vi "SelectOPCTags.HandleSymbolSelection.vi"(7 "This VI":refnum<vi>, 8 "error in":errorcluster, 10 "Tag":string, 11 "CtlRef":refnum<vi>) -> (0 "error out":errorcluster)   [LabVIEW 2015, in "OPC UA Client System Explorer.lvlib"]
uses:
  OPC UA Client System Explorer.lvlib
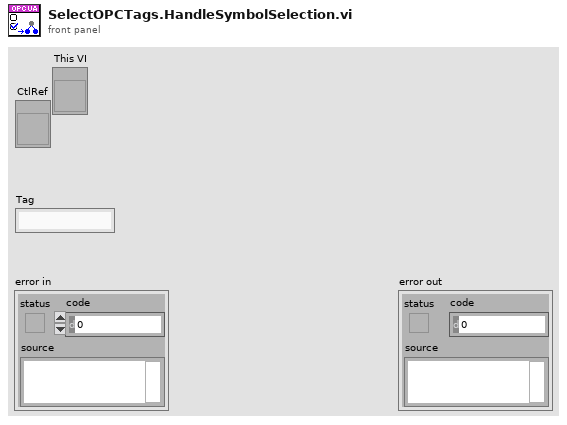
[diagram p1: front panel]
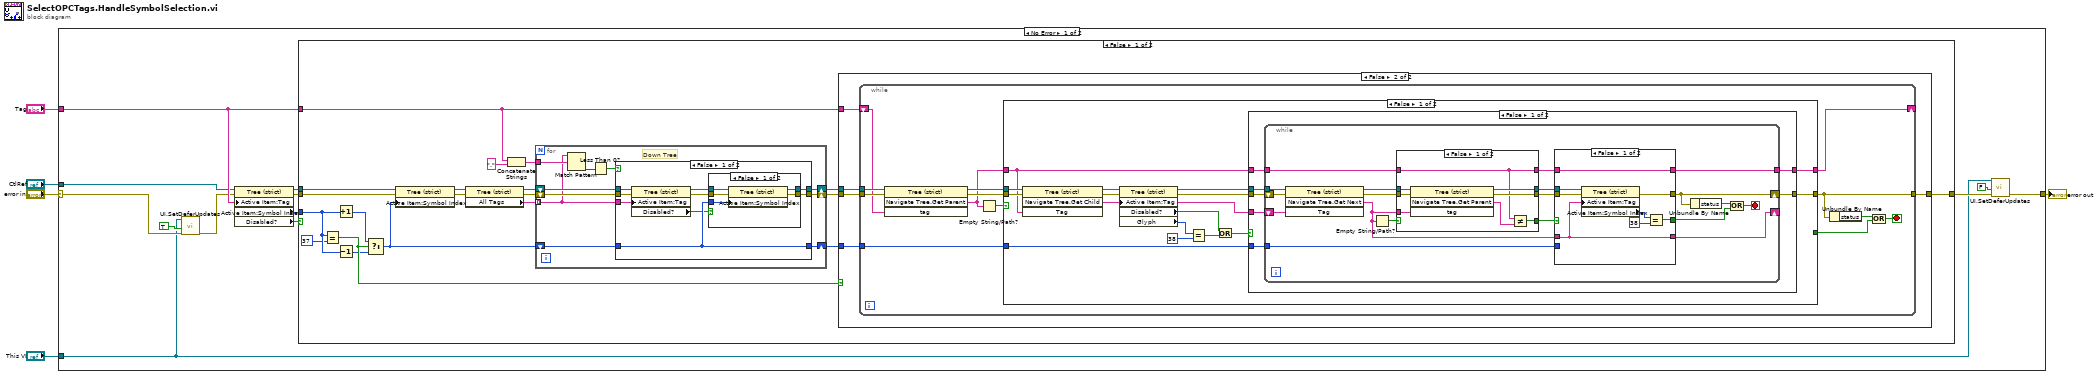
[diagram p0: block diagram]
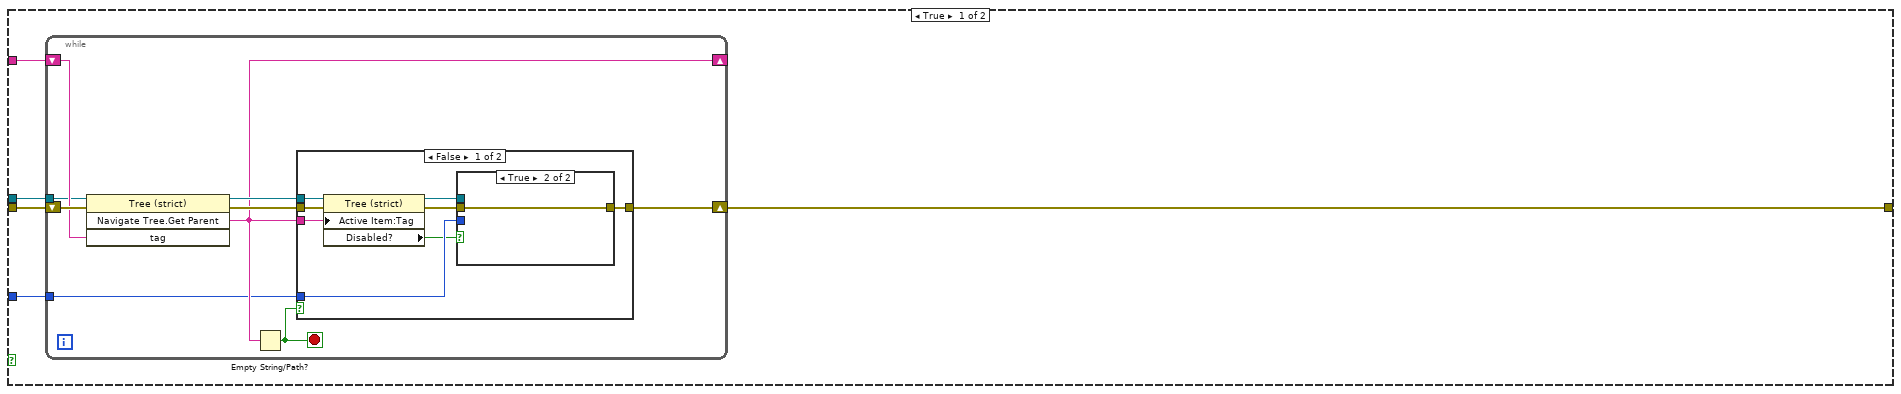
[diagram p2: hidden frame]
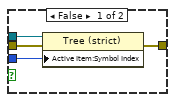
[diagram p3: hidden frame]
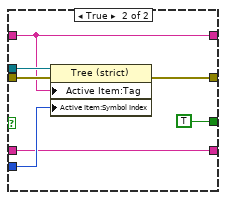
[diagram p6: hidden frame]
diagram:
  n1 = case shown="No Error" "error in" {
    selector: "error in" -> [w11 w189]
    tunnel: [w8 w189] -> w5
    tunnel: "Tag" -> [w18 _]
    tunnel: "CtlRef" -> [w17 _]
    tunnel: "This VI" -> [w6 _]
    frame No Error {
      n2 = call "UI.SetDeferUpdates.vi"("error in (no error)"=w11, "Defer Panel Updates"=TRUE, "This VI"=w6) -> ("error out"=w10:errorcluster)  [unwired: 8 in]
      n3 = property class="Tree (strict)"(reference=w17, error in=w10, "Active Item:Tag"=w18) -> (reference out=w15:refnum<vi>, error out=w16:errorcluster, "Active Item:Symbol Index"=w14:i32, "Disabled?"=w13:bool)
      n4 = case shown="False" w13 {
        tunnel: [w37 w188] -> w7
        tunnel: w18 -> [w35 _]
        tunnel: w16 -> [w24 w188]
        tunnel: w15 -> [w23 _]
        tunnel: w14 -> [w21 _]
        frame False {
          n5 = Equal?(x=w21, y=37 ("Active Item:Symbol Index")) -> (x = y?=w32:bool)
          n6 = Increment(x=w21) -> (x+1=w20:i32)
          n7 = Decrement(x=w21) -> (x-1=w22:i32)
          n8 = Select(t=w20, s=w32, f=w22) -> (s? t:f=w33:i32)
          n9 = property class="Tree (strict)"(reference=w23, error in=w24, "Active Item:Symbol Index"=w33) -> (reference out=w25:refnum<vi>, error out=w26:errorcluster)
          n10 = property class="Tree (strict)"(reference=w25, error in=w26) -> (reference out=w28:refnum<vi>, error out=w27:errorcluster, "All Tags"=w31:string[])
          n11 = Concatenate Strings(w35, "." ("string")) -> (w30:string)
          n12 = for {
            tunnel: w30 -> [w168]
            tunnel: w31 -> [w161] mode=indexing
            shift-right: [w164] -> w34
            shift-left: w27 -> [w163]
            shift-right: [w160] -> w36
            shift-left: w28 -> [w162]
            shift-right: [w159] -> w38
            shift-left: w33 -> [w165]
            # "Down Tree"
            n13 = Match Pattern(string=w161, regular expression=w168) -> (offset past match=w167:i32)  [unwired: 1 in, 3 out]
            n14 = Less Than 0?(x=w167) -> (x < 0?=w166:bool)
            n15 = case shown="False" w166 {
              tunnel: w163 -> [w176 w187]
              tunnel: w162 -> [w177 w186]
              tunnel: w161 -> [w175 _]
              tunnel: w165 -> [w170 w185]
              tunnel: [w171 w187] -> w164
              tunnel: [w172 w186] -> w160
              tunnel: [w170 w185] -> w159
              frame False {
                n16 = property class="Tree (strict)"(reference=w177, error in=w176, "Active Item:Tag"=w175) -> (reference out=w173:refnum<vi>, error out=w174:errorcluster, "Disabled?"=w169:bool)
                n17 = case shown="False" w169 {
                  tunnel: w174 -> [w182 w183]
                  tunnel: w173 -> [w181 w184]
                  tunnel: [w180 w184] -> w172
                  tunnel: [w179 w183] -> w171
                  tunnel: w170 -> [w178 _]
                  frame False {
                    n18 = property class="Tree (strict)"(reference=w181, error in=w182, "Active Item:Symbol Index"=w178) -> (reference out=w180:refnum<vi>, error out=w179:errorcluster)
                  }
                  frame True {
                  }
                }
              }
              frame True {
              }
            }
          }
          n19 = case shown="False" w32 {
            tunnel: w34 -> [w43 w70]
            tunnel: w35 -> [w42 w68]
            tunnel: w36 -> [w41 w69]
            tunnel: [w40 w71] -> w37
            tunnel: w38 -> [w39 w67]
            frame True {
              n20 = while {
                tunnel: w41 -> [w50]
                shift-right: [w45] -> w40
                shift-left: w43 -> [w52]
                shift-right: [w47] -> _
                shift-left: w42 -> [w51]
                tunnel: w39 -> [w46]
                stop <- w44 stop-if-true
                n21 = invoke on="Invoke Node" class="Tree (strict)" method="Navigate Tree.Get Parent"(reference=w50, error in=w52, "tag"=w51) -> (reference out=w49:refnum<vi>, error out=w48:errorcluster, "Navigate Tree:Get Parent"=w47:string)  [unwired: 1 in, 1 out]
                n22 = Empty String/Path?(string/path=w47) -> (empty?=w44:bool)
                n23 = case shown="False" w44 {
                  tunnel: w48 -> [w59 w66]
                  tunnel: w49 -> [w60 _]
                  tunnel: w47 -> [w58 _]
                  tunnel: w46 -> [w54 _]
                  tunnel: [w55 w66] -> w45
                  frame False {
                    n24 = property class="Tree (strict)"(reference=w60, error in=w59, "Active Item:Tag"=w58) -> (reference out=w56:refnum<vi>, error out=w57:errorcluster, "Disabled?"=w53:bool)
                    n25 = case shown="True" w53 {
                      tunnel: w57 -> [w64 w65]
                      tunnel: w56 -> [w63 _]
                      tunnel: [w62 w65] -> w55
                      tunnel: w54 -> [w61 _]
                      frame False {
                        n26 = property class="Tree (strict)"(reference=w63, error in=w64, "Active Item:Symbol Index"=w61) -> (error out=w62:errorcluster)  [unwired: 1 out]
                      }
                      frame True {
                      }
                    }
                  }
                  frame True {
                  }
                }
              }
            }
            frame False {
              n27 = while {
                tunnel: [w75] -> w71
                tunnel: w70 -> [w84]
                tunnel: w69 -> [w83]
                shift-right: [w78] -> _
                shift-left: w68 -> [w77]
                tunnel: w67 -> [w76]
                stop <- w73 stop-if-true
                n28 = invoke on="Invoke Node" class="Tree (strict)" method="Navigate Tree.Get Parent"(reference=w83, error in=w84, "tag"=w77) -> (reference out=w81:refnum<vi>, error out=w82:errorcluster, "Navigate Tree:Get Parent"=w80:string)  [unwired: 1 in, 1 out]
                n29 = Empty String/Path?(string/path=w80) -> (empty?=w79:bool)
                n30 = case shown="False" w79 {
                  selector: w79 -> [_ w156]
                  tunnel: w76 -> [w100 _]
                  tunnel: [w99 w158] -> w75
                  tunnel: w82 -> [w98 w158]
                  tunnel: w81 -> [w97 _]
                  tunnel: w80 -> [w92 w157]
                  tunnel: [w90 w157] -> w78
                  tunnel: [_ w156] -> w72
                  frame False {
                    n31 = invoke on="Invoke Node" class="Tree (strict)" method="Navigate Tree.Get Child"(reference=w97, error in=w98, "Tag"=w92) -> (reference out=w96:refnum<vi>, error out=w94:errorcluster, "Navigate Tree:Get Child"=w85:string)  [unwired: 1 in, 1 out]
                    n32 = property class="Tree (strict)"(reference=w96, error in=w94, "Active Item:Tag"=w85) -> (reference out=w95:refnum<vi>, error out=w93:errorcluster, "Disabled?"=w88:bool, "Glyph"=w89:i32)
                    n33 = Equal?(x=w89, y=38 ("Active Item:Symbol Index")) -> (x = y?=w87:bool)
                    n34 = Or(x=w88, y=w87) -> (x .or. y?=w86:bool)
                    n35 = case shown="False" w86 {
                      tunnel: w100 -> [w107 _]
                      tunnel: [w106 w155] -> w99
                      tunnel: w95 -> [w105 _]
                      tunnel: w93 -> [w104 w155]
                      tunnel: w85 -> [w103 _]
                      tunnel: w92 -> [w102 w154]
                      tunnel: [w101 w154] -> w90
                      frame False {
                        n36 = while {
                          tunnel: w107 -> [w126]
                          tunnel: w105 -> [w123]
                          shift-right: [w113] -> w106
                          shift-left: w104 -> [w125]
                          shift-right: [w108] -> _
                          shift-left: w103 -> [w124]
                          tunnel: w102 -> [w114]
                          tunnel: [w109] -> w101
                          stop <- w111 stop-if-true
                          n37 = invoke on="Invoke Node" class="Tree (strict)" method="Navigate Tree.Get Next"(reference=w123, error in=w125, "Tag"=w124) -> (reference out=w122:refnum<vi>, error out=w120:errorcluster, "Navigate Tree:Get Next Item"=w115:string)  [unwired: 1 in, 1 out]
                          n38 = Empty String/Path?(string/path=w115) -> (empty?=w117:bool)
                          n39 = case shown="False" w117 {
                            selector: w117 -> [_ w138]
                            tunnel: w122 -> [w134 w136]
                            tunnel: [w133 w136] -> w121
                            tunnel: w120 -> [w132 w137]
                            tunnel: [w131 w137] -> w119
                            tunnel: [w129 w138] -> w118
                            tunnel: w114 -> [w127 w135]
                            tunnel: w115 -> [w128 _]
                            tunnel: [w127 w135] -> w116
                            frame False {
                              n40 = invoke on="Invoke Node" class="Tree (strict)" method="Navigate Tree.Get Parent"(reference=w134, error in=w132, "tag"=w128) -> (reference out=w133:refnum<vi>, error out=w131:errorcluster, "Navigate Tree:Get Parent"=w130:string)  [unwired: 1 in, 1 out]
                              n41 = Not Equal?(x=w127, y=w130) -> (x != y?=w129:bool)
                            }
                            frame True {
                            }
                          }
                          n42 = case shown="False" w118 {
                            tunnel: w126 -> [_ w149]
                            tunnel: w119 -> [w146 w151]
                            tunnel: [w141 w152] -> w113
                            tunnel: w121 -> [w145 w150]
                            tunnel: w115 -> [w139 w147]
                            tunnel: [w142 TRUE] -> w110
                            tunnel: w116 -> [w140 w148]
                            tunnel: [w140 w148] -> w109
                            tunnel: [w139 w147] -> w108
                            frame False {
                              n43 = property class="Tree (strict)"(reference=w145, error in=w146, "Active Item:Tag"=w139) -> (error out=w141:errorcluster, "Active Item:Symbol Index"=w143:i32)  [unwired: 1 out]
                              n44 = Equal?(x=w143, y=38 ("Active Item:Symbol Index")) -> (x = y?=w142:bool)
                            }
                            frame True {
                              n45 = property class="Tree (strict)"(reference=w150, error in=w151, "Active Item:Tag"=w148, "Active Item:Symbol Index"=w149) -> (error out=w152:errorcluster)  [unwired: 1 out]
                            }
                          }
                          n46 = Unbundle By Name(w113) -> ("status"=w112:bool)
                          n47 = Compound Arithmetic op=OR(w112, w110) -> (w111:bool)
                        }
                      }
                      frame True {
                      }
                    }
                  }
                  frame True {
                  }
                }
                n48 = Unbundle By Name(w75) -> ("status"=w74:bool)
                n49 = Compound Arithmetic op=OR(w74, w72) -> (w73:bool)
              }
            }
          }
        }
        frame True {
        }
      }
      n50 = call "UI.SetDeferUpdates.vi"("error in (no error)"=w7, "Defer Panel Updates"=FALSE, "This VI"=w6) -> ("error out"=w8:errorcluster)  [unwired: 8 in]
    }
    frame Error {
    }
  }
  "error out" <- w5
